vi "Grips Slave Bandwidth.vi"() -> ()   [LabVIEW 2013]
uses:
  Telemanipulation/PXI/PXI.lvclass
  Telemanipulation/Grips Robot/Grips Robot.lvclass
  labview_ros/osrf_msgs/JointCommands.ctl
  <vilib>/platform/TimedLoop/XDataNode/XDataNode.xnode
  <vilib>/Platform/TimedLoop/XDataNode/nitl_modes.ctl
  <vilib>/Platform/TimedLoop/XDataNode/XDNodeRunTimeDep.lvlib
  <vilib>/Platform/TimedLoop/XDataNode/wakeup.ctl
  <vilib>/Platform/TimedLoop/XDataNode/timing_clust.ctl
  <userlib>/_matio/level5.lvlib
  Telemanipulation/Helpers/Helpers.lvlib
  <vilib>/ptbypt/NI_PtbyPt.lvlib
  <userlib>/_matio/level5/Public/Write/Append Data Element.llb/Append Data Element (2D Array of Double).vi
  <userlib>/_matio/level5/Public/Write/Append Data Element.llb/Append Data Element (1D Array of Double).vi
panel:
  in  "amplitude":dbl=0.05 min=0.0 max=1.0 step=0.05
  in  "joint":enum16{"SA", "SE", "EL", "WP", "WY", "WR"}(ring)=enum."WR"
  in  "Gen Sine":bool
  in  "frequency":dbl=10.0 min=0.0 max=20.0 step=0.5
  in  "Data Logging":cluster{"Path":path, "Save":bool}={"Path"=path "c:/ni-rt/fsuarez/wr_bandwidth.mat", "Save"=FALSE}
  out "Logging Status":errorcluster
  out "Joint Names":string[](array[string])=["SA", "SE", "EL", "WP", "WY", "WR"]
  in  "WR":dbl(slide)=-0.8744864101321355 scale=-3.14..3.14
  in  "WY":dbl(slide)=0.14750884043077422 scale=-1.01..0.67
  in  "WP":dbl(slide)=-0.4272375377563565 scale=-0.58..1.1
  in  "EL":dbl(slide)=3.14865864320094 scale=0.74..4.2
  in  "SE":dbl(slide)=-1.0575738697647323 scale=-1.5..0.5
  in  "SA":dbl(slide)=0.24276423851477275 scale=-1.5..1.5
  in  "Hyd ON":bool
  in  "kp_position":dbl[](array[numeric])=[3.0, -1.5, 2.0, 4.0, -2.0, 4.0]
  in  "stop":bool
  out "System Status":errorcluster
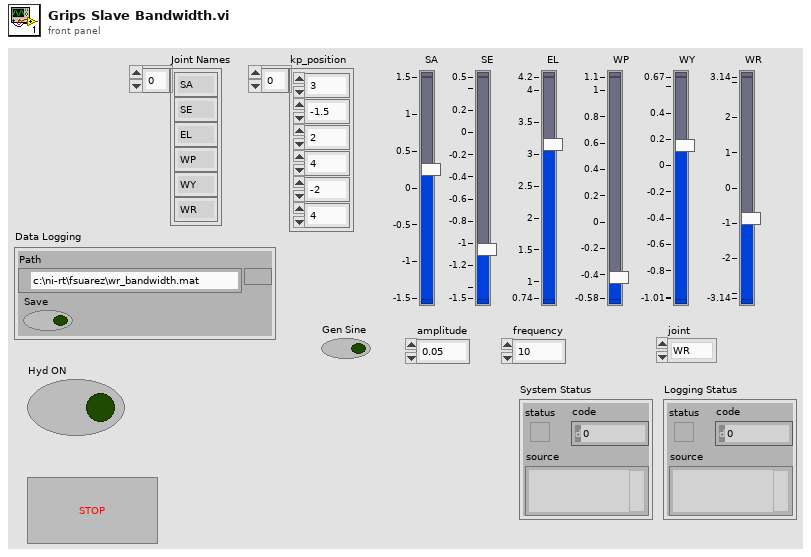
[diagram p1: front panel]
types:
  T1 = typedef "XDNodeRunTimeDep.lvlib/timing_clust.ctl" = cluster{"Expected End [f-1]":u64, "Actual End [f-1]":u64, "Finished Late? [f-1]":bool, "Expected End [i-1]":u64, "Actual End [i-1]":u64, "Finished Late? [i-1]":bool, "Expected Start [i]":u64, "Actual Start [i]":u64, "Expected Start [f]":u64, "Actual Start [f]":u64, "Source Name":string, "Structure Name":string, "Period":i64, "Deadline":i64, "Offset":i64, "Start":i64, "Priority":i32, "Timeout":i32, "Mode":T2, "Wakeup Reason":T3, "Error":errorcluster, "Source Type":string, "Secondary Source Type":string, "Global End Time":u64, "Global Start Time":u64, "Frame Duration":u64, "Iteration Duration":u64, "Assigned CPU":i32, "I/O Scan Engine Mode":u32}
  T2 = typedef "XDNodeRunTimeDep.lvlib/nitl_modes.ctl" = enum32{"No Change", "Process missed periods, maintain original phase", "Discard missed periods, maintain original phase", "Process missed periods, ignore original phase", "Discard missed periods, ignore original phase"}
  T3 = typedef "XDNodeRunTimeDep.lvlib/wakeup.ctl" = enum32{"Normal", "Aborted", "Asynchronous wakeup", "Timing source error", "Timed loop error", "Timeout"}
  T4 = typedef "Grips Robot.lvclass/JointMapping.ctl" = cluster{"name":string[], "position":string[], "velocity":string[], "effort":string[], "command":string[]}
  T5 = cluster{"names":cluster{"AI":string[], "AO":string[], "DI":string[], "DO":string[]}, "interpolation_coeff":sgl[][]}
  T6 = typedef "NI_Robotics_Link.lvclass/Joint Type.ctl" = enum16{"Revolute", "Prismatic"}
  T7 = cluster{"k":sgl[][], "p":sgl[][], "T0":sgl[][], "types":T6[], "joint_limits":cluster{"has_limits":bool[], "min_position":sgl[], "max_position":sgl[]}}
  T8 = cluster{"AI":string[], "AO":string[], "DI":string[], "DO":string[]}
  T9 = typedef "PXI.lvclass/Task Definition.ctl" = cluster{"task_type":T10, "names":string[], "physical channels":tag, "min_value":dbl, "max_value":dbl, "task_number":i32}
  T10 = typedef "PXI.lvclass/Task Types.ctl" = enum16{"Analog Input", "Analog Output", "Digital Input", "Digital Output"}
  T11 = enum16{"open", "replace", "create", "open or create", "replace or create", "replace or create with confirmation"}
  T12 = typedef "Hardware Interface.lvclass/BoolArrayWithName.ctl" = cluster{"name":string[], "value":bool[]}
  T13 = typedef "Hardware Interface.lvclass/DblArrayWithName.ctl" = cluster{"name":string[], "value":dbl[]}
  T14 = typedef "JointState.ctl" = cluster{"header":cluster{"seq":u32, "stamp":cluster{"sec":i32, "nsec":i32}, "frame_id":string}, "name":string[], "position":dbl[], "velocity":dbl[], "effort":dbl[]}
  T15 = typedef "JointCommands.ctl" = cluster{"header":cluster{"seq":u32, "stamp":cluster{"sec":i32, "nsec":i32}, "frame_id":string}, "name":string[], "position":dbl[], "velocity":dbl[], "effort":dbl[], "kp_position":dbl[], "ki_position":dbl[], "kd_position":dbl[], "kp_velocity":dbl[], "i_effort_min":dbl[], "i_effort_max":dbl[]}
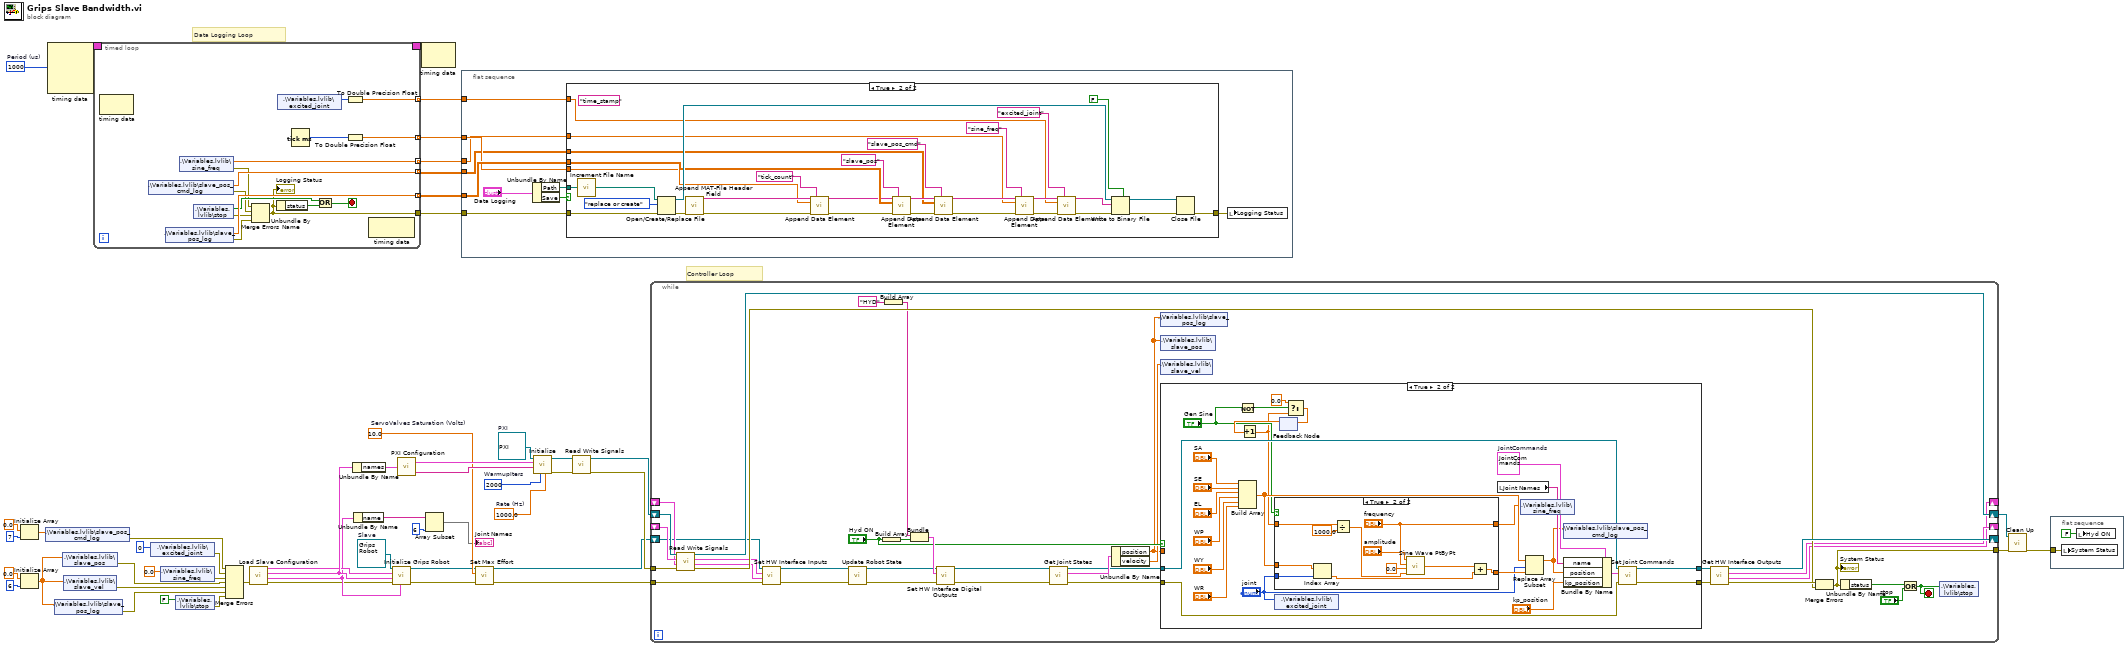
[diagram p0: block diagram]
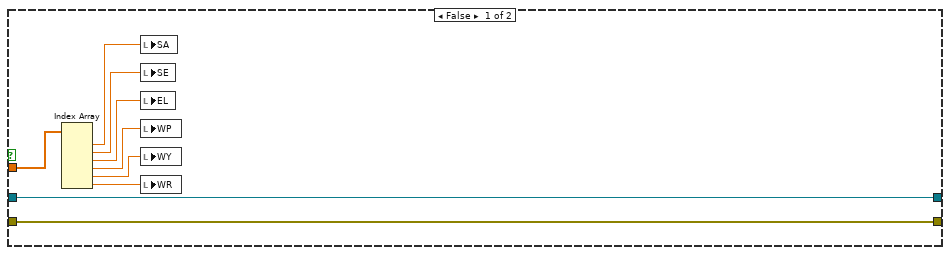
[diagram p3: hidden frame]
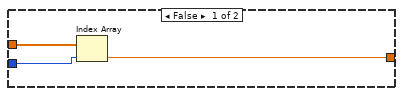
[diagram p4: hidden frame]
diagram:
  w10 = i64 1000  # Period (us)
  w36 = 10.0  # ServoValves Saturation (Volts)
  w39 = refnum<class "Grips Robot.lvclass"> refnum  # Slave
  w50 = 1000.0  # Rate (Hz)
  w51 = u32 2000  # WarmupIters
  w52 = refnum<class "PXI.lvclass"> refnum  # PXI
  # "Data Logging Loop"
  # "Controller Loop"
  n1 = Initialize Array(0.0 ("element"), 7 ("dimension size")) -> (w9:dbl[])
  n2 = Initialize Array(0.0 ("element"), 6 ("dimension size")) -> (w16:dbl[])
  n3 = shared-variable ".\\Variables.lvlib\\slave_pos_cmd_log"(w9) -> (error out=w1:errorcluster)  [unwired: 1 in]
  n4 = node-c288(w10) -> (w19:T1)  [unwired: 3 in]
  n5 = shared-variable ".\\Variables.lvlib\\slave_pos_log"(w16) -> (error out=w15:errorcluster)  [unwired: 1 in]
  n6 = shared-variable ".\\Variables.lvlib\\slave_pos"(w16) -> (error out=w31:errorcluster)  [unwired: 1 in]
  n7 = shared-variable ".\\Variables.lvlib\\slave_vel"(w16) -> (error out=w30:errorcluster)  [unwired: 1 in]
  n8 = timed-loop {
    timing: w19 -> [_]
    timing-out: [_] -> w18
    tunnel: [w67] -> w13 mode=indexing
    tunnel: [w65] -> w12 mode=indexing
    tunnel: [w55] -> w11
    tunnel: [w61] -> w8 mode=indexing
    tunnel: [w60] -> w5 mode=indexing
    tunnel: [w53] -> w2 mode=indexing
    stop <- w62 stop-if-true
    n9 = node-c288() -> ()  [unwired: 1 in, 1 out]
    n10 = shared-variable ".\\Variables.lvlib\\slave_pos_cmd_log"() -> (w61:dbl[], error out=w58:errorcluster)  [unwired: 1 in]
    n11 = shared-variable ".\\Variables.lvlib\\slave_pos_log"() -> (w67:dbl[], error out=w56:errorcluster)  [unwired: 1 in]
    n12 = shared-variable ".\\Variables.lvlib\\sine_freq"() -> (w60:dbl, error out=w59:errorcluster)  [unwired: 1 in]
    n13 = shared-variable ".\\Variables.lvlib\\stop"() -> (w63:bool, error out=w57:errorcluster)  [unwired: 1 in]
    n14 = Merge Errors(w59, w58, w57, w56) -> (w55:errorcluster)
    "Logging Status" <- w55
    n15 = Unbundle By Name(w55) -> ("status"=w64:bool)
    n16 = shared-variable ".\\Variables.lvlib\\excited_joint"() -> (w54:u16)  [unwired: 1 in, 1 out]
    n17 = Tick Count (ms)() -> (millisecond timer value=w66:u32)
    n18 = Or(x=w63, y=w64) -> (x .or. y?=w62:bool)
    n19 = To Double Precision Float(number=w54) -> (double precision float=w53:dbl)
    n20 = To Double Precision Float(number=w66) -> (double precision float=w65:dbl)
    n21 = node-c288() -> ()  [unwired: 1 in, 1 out]
  }
  n22 = shared-variable ".\\Variables.lvlib\\excited_joint"(u16 0 ("excited_joint")) -> (error out=w3:errorcluster)  [unwired: 1 in]
  n23 = shared-variable ".\\Variables.lvlib\\sine_freq"(0.0 ("sine_freq")) -> (error out=w6:errorcluster)  [unwired: 1 in]
  n24 = shared-variable ".\\Variables.lvlib\\stop"(FALSE ("stop")) -> (error out=w14:errorcluster)  [unwired: 1 in]
  n25 = Merge Errors(w1, w3, w6, w31, w30, w15, w14) -> (w17:errorcluster)
  n26 = call "Load Slave Configuration.vi"("error in"=w17) -> ("error out"=w20:errorcluster, "JointMapping"=w25:T4, "hw interface"=w38:T5, "kinematic parameters"=w37:T7)  [unwired: 7 in]
  n27 = Unbundle By Name(w38) -> ("names"=w40:T8)
  n28 = Unbundle By Name(w25) -> ("name"=w24:string[])
  n29 = call "Initialize Grips Robot.vi"("JointMapping"=w25, "error in (no error)"=w20, "hw interface"=w38, "kinematic_parameters"=w37, "Grips Robot in"=w39) -> ("error out"=w33:errorcluster, "Grips Robot out"=w34:refnum<class "Grips Robot.lvclass">)  [unwired: 5 in]
  n30 = call "PXI Configuration.vi"("names"=w40) -> ("Master Clock"=w41:tag, "Tasks Configuration"=w42:T9[])  [unwired: 2 in]
  n31 = node-c288(w18) -> ()  [unwired: 1 out]
  n32 = Array Subset(array=w24, length=6) -> (→"Joint Names":string[])  [unwired: 1 in]
  n33 = flat-sequence {
    tunnel: w13 -> [w78]
    tunnel: w12 -> [w77]
    tunnel: w11 -> [w73]
    tunnel: w8 -> [w72]
    tunnel: w5 -> [w71]
    tunnel: w2 -> [w70]
    frame #0 {
      n34 = Unbundle By Name("Data Logging") -> ("Path"=w75:path, "Save"=w74:bool)
      n35 = case shown="True" w74 {
        tunnel: [w80 w103] -> w79
        tunnel: w78 -> [_ w102]
        tunnel: w77 -> [_ w101]
        tunnel: w75 -> [_ w95]
        tunnel: w73 -> [w80 w97]
        tunnel: w72 -> [_ w92]
        tunnel: w71 -> [_ w87]
        tunnel: w70 -> [_ w82]
        frame False {
        }
        frame True {
          (unwired) "time_stamp" ("Data Name")
          n36 = call "Increment File Name.vi"("Full Path"=w95) -> ("New Path"=w96:path)
          n37 = Open/Create/Replace File(file path (use dialog)=w96, error in=w97, operation (0:open)=T11."replace or create") -> (refnum out=w104:refnum<file>, error out=w100:errorcluster)  [unwired: 3 in, 1 out]
          n38 = call <userlib>:"Append MAT-File Header Field.vi"("error"=w100) -> ("result string"=w108:string, "error out"=w107:errorcluster)  [unwired: 13 in]
          n39 = call-poly <userlib>:"Append Data Element.vi"("initial string"=w108, "Data Name"="tick_count", "data"=w101, "error in"=w107) -> ("result string"=w99:string, "error out"=w98:errorcluster)  [unwired: 10 in]
          n40 = call-poly <userlib>:"Append Data Element.vi"("initial string"=w99, "Data Name"="slave_pos" ("array name"), "data"=w102, "error in"=w98) -> ("result string"=w94:string, "error out"=w93:errorcluster)  [unwired: 10 in]
          n41 = call-poly <userlib>:"Append Data Element.vi"("initial string"=w94, "Data Name"="slave_pos_cmd" ("array name"), "data"=w92, "error in"=w93) -> ("result string"=w89:string, "error out"=w90:errorcluster)  [unwired: 10 in]
          n42 = call-poly <userlib>:"Append Data Element.vi"("initial string"=w89, "Data Name"="sine_freq", "data"=w87, "error in"=w90) -> ("result string"=w83:string, "error out"=w86:errorcluster)  [unwired: 10 in]
          n43 = call-poly <userlib>:"Append Data Element.vi"("initial string"=w83, "Data Name"="excited_joint", "data"=w82, "error in"=w86) -> ("result string"=w84:string, "error out"=w85:errorcluster)  [unwired: 10 in]
          n44 = Write to Binary File(file (use dialog)=w104, data=w84, error in=w85, 5:FALSE ("prepend array or string size? (T)")) -> (refnum out=w110:refnum<file>, error out=w109:errorcluster)  [unwired: 2 in, 1 out]
          n45 = Close File(refnum=w110, error in=w109) -> (error out=w103:errorcluster)  [unwired: 1 out]
        }
      }
      n46 = local write "Logging Status"(w79) -> ()
    }
  }
  n47 = call "Set Max Effort.vi"("error in (no error)"=w33, "max effort"=w36, "Grips Robot in"=w34) -> ("error out"=w35:errorcluster, "Grips Robot out"=w32:refnum<class "Grips Robot.lvclass">)  [unwired: 7 in]
  n48 = call "Initialise.vi"("Rate (Hz)"=w50, "WarmupIters"=w51, "Master Clock"=w41, "Tasks Config"=w42, "PXI in"=w52) -> ("error out"=w48:errorcluster, "PXI out"=w49:refnum<class "PXI.lvclass">)  [unwired: 5 in]
  n49 = call "Read Write Signals.vi"("error in (no error)"=w48, "PXI in"=w49) -> ("error out"=w46:errorcluster, "PXI out"=w47:refnum<class "PXI.lvclass">)  [unwired: 6 in, 2 out]
  n50 = while {
    shift-right: [w146] -> w45
    shift-left: w47 -> [w147]
    tunnel: w46 -> [w148]
    tunnel: [w139] -> w44
    tunnel: w35 -> [w143]
    shift-right: [w135] -> _
    shift-left: _ -> [w136]
    shift-right: [w133] -> _
    shift-left: _ -> [w134]
    shift-right: [w142] -> _
    shift-left: w32 -> [w116]
    stop <- w115 stop-if-true
    n51 = call "Read Write Signals.vi"("error in (no error)"=w148, "Digital Outputs"=w134, "Analog Outputs"=w136, "PXI in"=w147) -> ("error out"=w140:errorcluster, "Digital Inputs"=w137:T12, "Analog Inputs"=w138:T13, "PXI out"=w146:refnum<class "PXI.lvclass">)  [unwired: 4 in]
    n52 = call "Set HW Interface Inputs.vi"("error in (no error)"=w143, "Digital Inputs"=w137, "Analog Inputs"=w138, "Grips Robot in"=w116) -> ("error out"=w131:errorcluster, "Grips Robot out"=w132:refnum<class "Grips Robot.lvclass">)  [unwired: 6 in]
    n53 = call "Update Robot State.vi"("error in (no error)"=w131, "Grips Robot in"=w132) -> ("error out"=w117:errorcluster, "Grips Robot out"=w118:refnum<class "Grips Robot.lvclass">)  [unwired: 8 in]
    n54 = Build Array("Hyd ON") -> (w121:bool[])
    n55 = Build Array("HYD") -> (w120:string[])
    n56 = Bundle(w120, w121) -> (w123:cluster{string[], bool[]})  [unwired: 1 in]
    n57 = call "Set HW Interface Digital Outputs.vi"("error in (no error)"=w117, "Digital Outputs"=w123, "Grips Robot in"=w118) -> ("error out"=w124:errorcluster, "Grips Robot out"=w125:refnum<class "Grips Robot.lvclass">)  [unwired: 7 in]
    n58 = call "Get Joint States.vi"("error in (no error)"=w124, "Grips Robot in"=w125) -> ("error out"=w127:errorcluster, "JointState"=w130:T14, "Grips Robot out"=w129:refnum<class "Grips Robot.lvclass">)  [unwired: 7 in]
    n59 = Unbundle By Name(w130) -> ("position"=w113:dbl[], "velocity"=w114:dbl[])
    n60 = shared-variable ".\\Variables.lvlib\\slave_pos_log"(w113) -> ()  [unwired: 1 in, 1 out]
    n61 = shared-variable ".\\Variables.lvlib\\slave_pos"(w113) -> ()  [unwired: 1 in, 1 out]
    n62 = shared-variable ".\\Variables.lvlib\\slave_vel"(w114) -> ()  [unwired: 1 in, 1 out]
    n63 = case shown="True" "Hyd ON" {
      tunnel: w113 -> [w155 _]
      tunnel: w129 -> [w157 w171]
      tunnel: [w157 w180] -> w128
      tunnel: w127 -> [w156 w179]
      tunnel: [w156 w178] -> w126
      frame False {
        n64 = Index Array(array=w155) -> (element #1=w154:dbl, element #2=w153:dbl, element #3=w152:dbl, element #4=w151:dbl, element #5=w150:dbl, element #6=w149:dbl)  [unwired: 6 in]
        n65 = local write "SA"(w154) -> ()
        n66 = local write "SE"(w153) -> ()
        n67 = local write "EL"(w152) -> ()
        n68 = local write "WP"(w151) -> ()
        n69 = local write "WY"(w150) -> ()
        n70 = local write "WR"(w149) -> ()
      }
      frame True {
        w182 = T15 {"header"={"seq"=0, "stamp"={"sec"=0, "nsec"=0}, "frame_id"=""}, "name"=[], "position"=[], "velocity"=[], "effort"=[], "kp_position"=[], "ki_position"=[], "kd_position"=[], "kp_velocity"=[], "i_effort_min"=[], "i_effort_max"=[]}  # JointCommands
        n71 = Not(x="Gen Sine") -> (.not. x?=w159:bool)
        n72 = Build Array("SA", "SE", "EL", "WP", "WY", "WR") -> (w166:dbl[])
        n73 = shared-variable ".\\Variables.lvlib\\excited_joint"("joint") -> ()  [unwired: 1 in, 1 out]
        n74 = feedback #1() -> (w163:dbl)  [unwired: 1 in]
        n75 = Increment(x=w163) -> (x+1=w158:dbl)
        n76 = case shown="True" "Gen Sine" {
          tunnel: [w184 w194] -> w168
          tunnel: w166 -> [w185 w190]
          tunnel: "joint" -> [w183 w189]
          tunnel: [_ "frequency"] -> w165
          tunnel: w158 -> [_ w186]
          frame False {
            n77 = Index Array(array=w185, index=w183) -> (element=w184:dbl)
          }
          frame True {
            n78 = Index Array(array=w190, index=w189) -> (element=w188:dbl)
            n79 = Divide(x=w186, y=1000.0) -> (x/y=w193:dbl)
            n80 = call <vilib>:"Sine Wave PtByPt.vi"("time"=w193, "phase"=0.0, "frequency"="frequency", "amplitude"="amplitude") -> ("sine wave"=w195:dbl)
            n81 = Add(x=w195, y=w188) -> (x+y=w194:dbl)
          }
        }
        n82 = Select(t=0.0, s=w159, f=w158) -> (s? t:f=w162:dbl)
        n83 = feedback-in #1(w162) -> ()
        n84 = local read "Joint Names"() -> (w170:string[])
        n85 = shared-variable ".\\Variables.lvlib\\sine_freq"(w165) -> ()  [unwired: 1 in, 1 out]
        n86 = Replace Array Subset(array=w166, new element=w168, index="joint") -> (w167:dbl[])
        n87 = shared-variable ".\\Variables.lvlib\\slave_pos_cmd_log"(w167) -> ()  [unwired: 1 in, 1 out]
        n88 = Bundle By Name(cluster=w182, "name"=w170, "position"=w167, "kp_position"="kp_position") -> (w181:T15)
        n89 = call "Set Joint Commands.vi"("error in (no error)"=w179, 10:w181, "Grips Robot in"=w171) -> ("error out"=w178:errorcluster, "Grips Robot out"=w180:refnum<class "Grips Robot.lvclass">)  [unwired: 7 in]
      }
    }
    n90 = call "Get HW Interface Outputs.vi"("error in (no error)"=w126, "Grips Robot in"=w128) -> ("error out"=w141:errorcluster, "Digital Outputs"=w133:T12, "Analog Outputs"=w135:T13, "Grips Robot out"=w142:refnum<class "Grips Robot.lvclass">)  [unwired: 6 in]
    n91 = Merge Errors(w141, w140) -> (w139:errorcluster)
    "System Status" <- w139
    n92 = Unbundle By Name(w139) -> ("status"=w145:bool)
    n93 = Or(x=w145, y="stop") -> (x .or. y?=w115:bool)
    n94 = shared-variable ".\\Variables.lvlib\\stop"(w115) -> ()  [unwired: 1 in, 1 out]
  }
  n95 = call "Clean Up.vi"("error in (no error)"=w44, "PXI in"=w45) -> ("error out"=w43:errorcluster)  [unwired: 8 in, 1 out]
  n96 = flat-sequence {
    tunnel: w43 -> [w198]
    frame #0 {
      n97 = local write "System Status"(w198) -> ()
      n98 = local write "Hyd ON"(FALSE ("Hyd ON")) -> ()
    }
  }
